vi "Set Bitstream Mode.vi"(8 "error in":errorcluster, 10 "Bitstream mode (F)":bool, 11 "GOLPI ref. in":T1={"pipe handle"={"lv_proc.dll file path"=path "", "process instance handle"=[], "debug mode"=FALSE, "debug data"=[]}, "fast read timeout [ms]"=500, "fast read settle time [ms]"=10, "fast read to multiple [ms]"=1, "max elements per input line"=100, "slow read timeout [ms]"=5000, "stdin double format specifier"="", "max elements per stdout output column"=100, "console mode bitstream"=FALSE, "bitstream first read timeout [ms]"=1000, "bitstream read timeout [ms]"=50, "struct transfer possible"=FALSE, "matlab mode"=FALSE}) -> (0 "error out":errorcluster, 3 "GOLPI ref. out":T1={"pipe handle"={"lv_proc.dll file path"=path "", "process instance handle"=[], "debug mode"=FALSE, "debug data"=[]}, "fast read timeout [ms]"=500, "fast read settle time [ms]"=10, "fast read to multiple [ms]"=1, "max elements per input line"=100, "slow read timeout [ms]"=5000, "stdin double format specifier"="", "max elements per stdout output column"=100, "console mode bitstream"=FALSE, "bitstream first read timeout [ms]"=1000, "bitstream read timeout [ms]"=50, "struct transfer possible"=FALSE, "matlab mode"=FALSE})   [LabVIEW 2020, in "GOLPI library.lvlib"]
doc: "Set bitstream mode (only for GNU Octave, for Matlab not supported/needed). When set, data are transfered from Octave to LabVIEW using golpi GNU Octave package. This package codes variables into a stream of bits so data can be transfered to LabVIEW very fast. First this VI tries to install GNU Octave package golpi. Than package is loaded and VI checks if function golpi_data2bits() is available in current GNU Octave instance. If not error error is generated.\n\n---\nGOLPI works only with lv_proc.dll library, which is part of vipm package or should be delivered together with packed library. Placement of this dll is selected in terminal of Start GNU Octave.vi."
uses:
  GOLPI library.lvlib
  GOLPI reference Type Def.ctl
  Pipe Handle.ctl
  Custom Error Codes Enum Type Def.vi
  <vilib>/regexp/Match Regular Expression.xnode
  LV Process library.lvlib
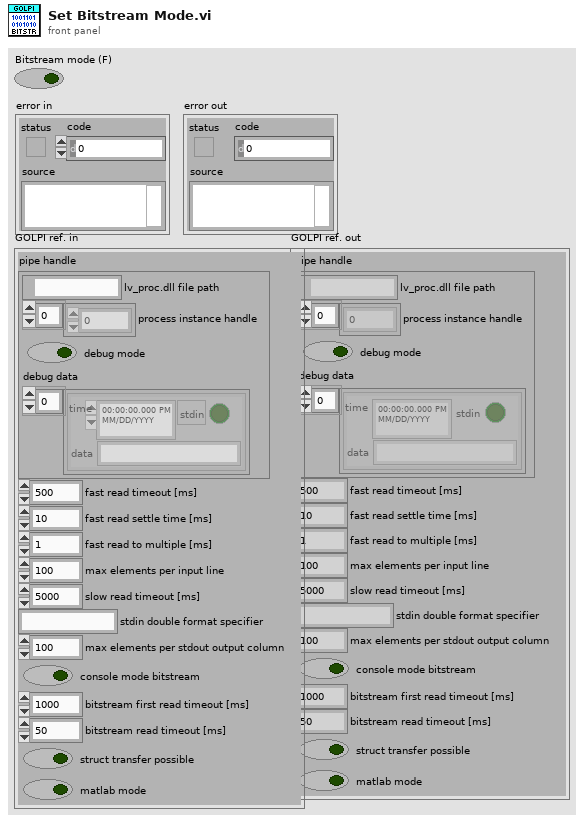
[diagram p1: front panel]
types:
  T1 = typedef "GOLPI library.lvlib/GOLPI reference Type Def.ctl" = cluster{"pipe handle":T2, "fast read timeout [ms]":u32, "fast read settle time [ms]":u32, "fast read to multiple [ms]":u32, "max elements per input line":u32, "slow read timeout [ms]":u32, "stdin double format specifier":string, "max elements per stdout output column":u32, "console mode bitstream":bool, "bitstream first read timeout [ms]":u32, "bitstream read timeout [ms]":u32, "struct transfer possible":bool, "matlab mode":bool}
  T2 = typedef "LV Process library.lvlib/Pipe Handle.ctl" = cluster{"lv_proc.dll file path":path, "process instance handle":u32[], "debug mode":bool, "debug data":cluster{"time":timestamp, "stdin":bool, "data":string}[]}
  T3 = typedef "GOLPI library.lvlib/Custom Error Codes Enum Type Def.vi" = enum16{"no error", "00 working directory PAR1 missing", "01 octave binary PAR1 missing", "02 octave report error PAR1", "03 empty output last cmd PAR1", "04 missing temporary file PAR1", "05 pwd PAR 1 not exist", "06 oct package not installed", "07 octave default binary missing", "10 var PAR1 not string, vect", "11 var PAR1 not num, scal, ~compl", "12 var PAR1 not num, scal, compl", "13 var PAR1 not num, vect, ~compl", "14 var PAR1 not num, vect, compl", "15 var PAR1 not num, mat, ~compl", "16 var PAR1 not num, mat, ~compl", "30 read timeout", "60 bitstream transport failed", "61 bitstream decode error PAR1", "62 bitstream cannot be set", "70 struct transfer not possible", "80 struct: cluster elem. PAR1 not implem.", "81 struct: structure field PAR1 not implem.", "82 struct: size mismatch of PAR1", "83 struct: type mismatch of PAR1", "98 internal error", "99 not finished", "90 Not supported in Matlab mode", "91 Matlab variable transfer error", "92 Matlab Script Error"}
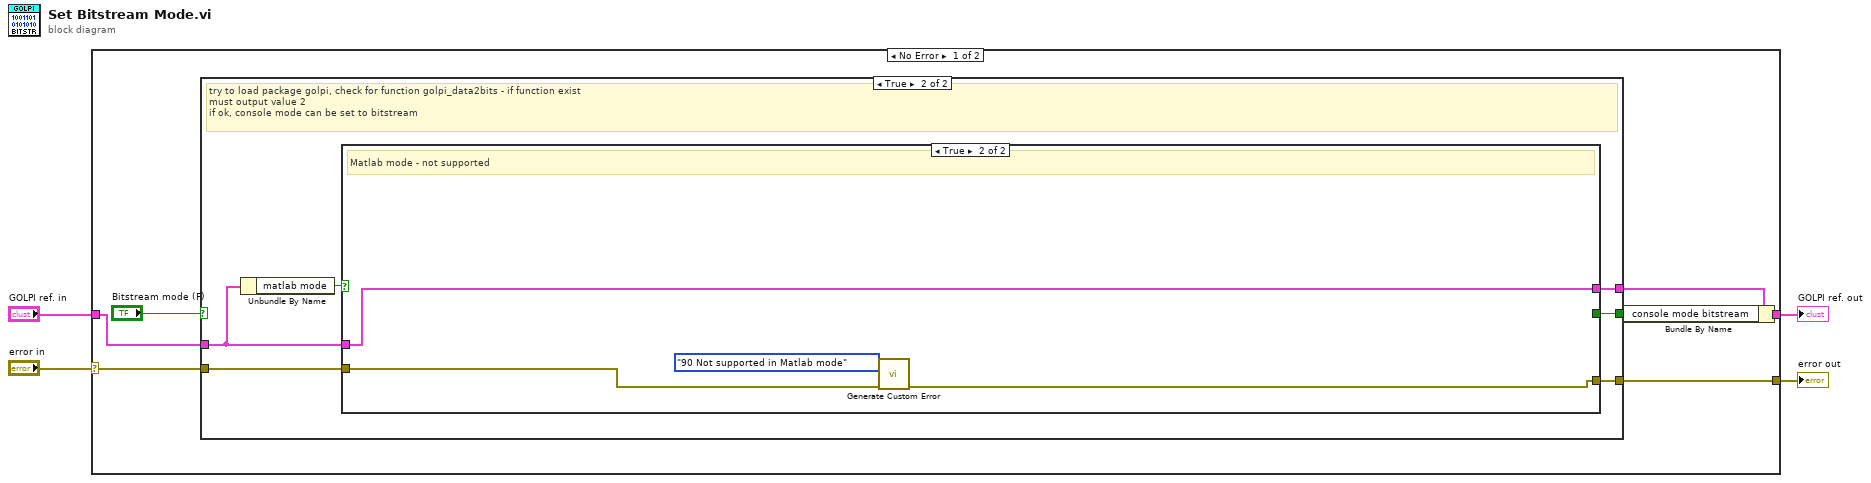
[diagram p0: block diagram]
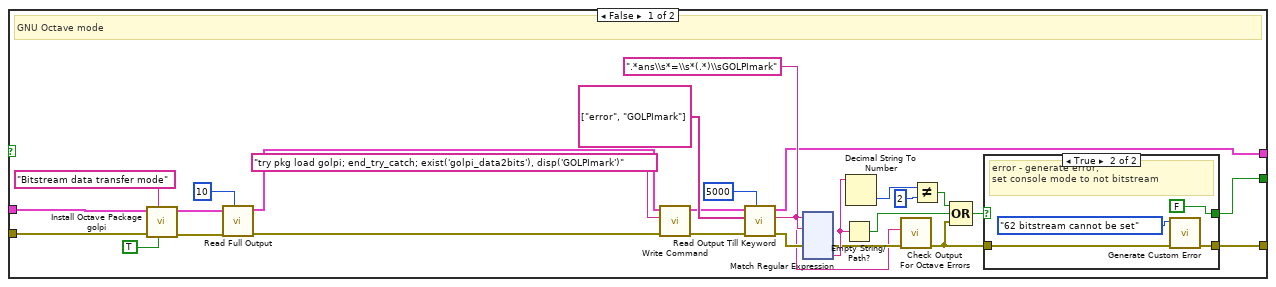
[diagram p3: hidden frame]
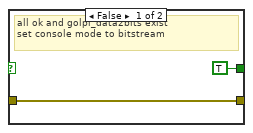
[diagram p4: hidden frame]
diagram:
  n1 = case shown="No Error" "error in" {
    selector: "error in" -> [w7 w176]
    tunnel: "GOLPI ref. in" -> [w8 w175]
    tunnel: [w11 w175] -> w3
    tunnel: [w6 w176] -> w1
    frame No Error {
      n2 = case shown="True" "Bitstream mode (F)" {
        selector: "Bitstream mode (F)" -> [w14 _]
        tunnel: [w14 w19] -> w9
        tunnel: w8 -> [w13 w16]
        tunnel: w7 -> [w12 w17]
        tunnel: [w12 w18] -> w6
        tunnel: [w13 w20] -> w5
        frame False {
          # "set console mode - this can be done withnout any checks or conditions"
        }
        frame True {
          # "try to load package golpi, check for function golpi_data2bits - if function exist\nmust output value 2\nif ok, console mode can be set to bitstream"
          n3 = Unbundle By Name(w16) -> ("matlab mode"=w15:bool)
          n4 = case shown="True" w15 {
            tunnel: [w35 w172] -> w20
            tunnel: [w32 _] -> w19
            tunnel: [w31 w171] -> w18
            tunnel: w17 -> [w26 w174]
            tunnel: w16 -> [w23 w172]
            frame False {
              # "GNU Octave mode"
              n5 = call "Install Octave Package golpi.vi"("Verbose? (T)"=TRUE, "Feature name"="Bitstream data transfer mode", "error in"=w26, "GOLPI ref. in"=w23) -> ("error out"=w25:errorcluster, "GOLPI ref. out"=w24:T1)  [unwired: 6 in]
              n6 = call "Read Full Output.vi"("timeout [ms]"=u32 10, "error in"=w25, "GOLPI ref. in"=w24) -> ("error out"=w47:errorcluster, "GOLPI ref. out"=w48:T1)  [unwired: 5 in, 2 out]
              n7 = call "Write Command.vi"("error in"=w47, "command"="try pkg load golpi; end_try_catch; exist('golpi_data2bits'), disp('GOLPImark')", "GOLPI ref. in"=w48) -> ("error out"=w38:errorcluster, "GOLPI ref. out"=w36:T1)  [unwired: 7 in]
              n8 = call "Read Output Till Keyword.vi"("timeout [ms]"=u32 5000, "error in"=w38, "keywords"=string[] ["error", "GOLPImark"], "GOLPI ref. in"=w36) -> ("error out"=w37:errorcluster, "read buffer"=w27:string, "GOLPI ref. out"=w35:T1)  [unwired: 4 in, 1 out]
              n9 = xnode "Match Regular Expression"("input string"=w27, "regular expression"=".*ans\\s*=\\s*(.*)\\sGOLPImark", "error in"=w37) -> ("error out"=w39:errorcluster, "submatch 1"=w42:string)  [unwired: 3 in, 4 out]
              n10 = Empty String/Path?(string/path=w42) -> (empty?=w43:bool)
              n11 = Decimal String To Number(string=w42) -> (number=w29:i32)  [unwired: 2 in, 1 out]
              n12 = call "Check Output For Octave Errors.vi"("error in"=w39, "read buffer"=w27) -> ("error out"=w28:errorcluster)  [unwired: 9 in]
              n13 = Not Equal?(x=w29, y=2) -> (x != y?=w40:bool)
              n14 = Compound Arithmetic op=OR(w40, w43, w28) -> (w33:bool)
              n15 = case shown="True" w33 {
                tunnel: [TRUE FALSE] -> w32
                tunnel: [w50 w52] -> w31
                tunnel: w28 -> [w50 w53]
                frame False {
                  # "all ok and golpi_data2bits exist\nset console mode to bitstream"
                }
                frame True {
                  # "error - generate error, \nset console mode to not bitstream"
                  n16 = call "Generate Custom Error.vi"("error in"=w53, "GOLPI error"=Custom_Error_Codes_Enum_Type_Def.vi."62 bitstream cannot be set") -> ("error out"=w52:errorcluster)  [unwired: 9 in]
                }
              }
            }
            frame True {
              # "Matlab mode - not supported"
              n17 = call "Generate Custom Error.vi"("error in"=w174, "GOLPI error"=Custom_Error_Codes_Enum_Type_Def.vi."90 Not supported in Matlab mode") -> ("error out"=w171:errorcluster)  [unwired: 9 in]
            }
          }
        }
      }
      n18 = Bundle By Name(cluster=w5, "console mode bitstream"=w9) -> (w11:T1)
    }
    frame Error {
    }
  }
  "error out" <- w1
  "GOLPI ref. out" <- w3
